vi "RX-SIM-BPCS-UDP (SubVI).vi"(8 "error in (no error)":errorcluster, 11 "UDP Network Connection in":refnum<k16>) -> (0 "error out":errorcluster, 1 "BPCS-10LI200":dbl, 2 "SIM-BPCS-RX-ARRAY":dbl[](array[numeric]), 3 "UDP Network Connection out":refnum<k16>, 5 "BPCS-10TI100":dbl)   [LabVIEW 2018]
uses:
  BPCS Global Variables.vi
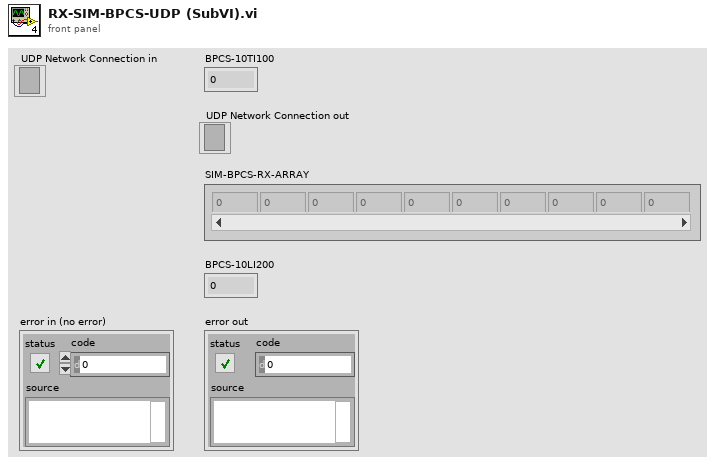
[diagram p1: front panel]
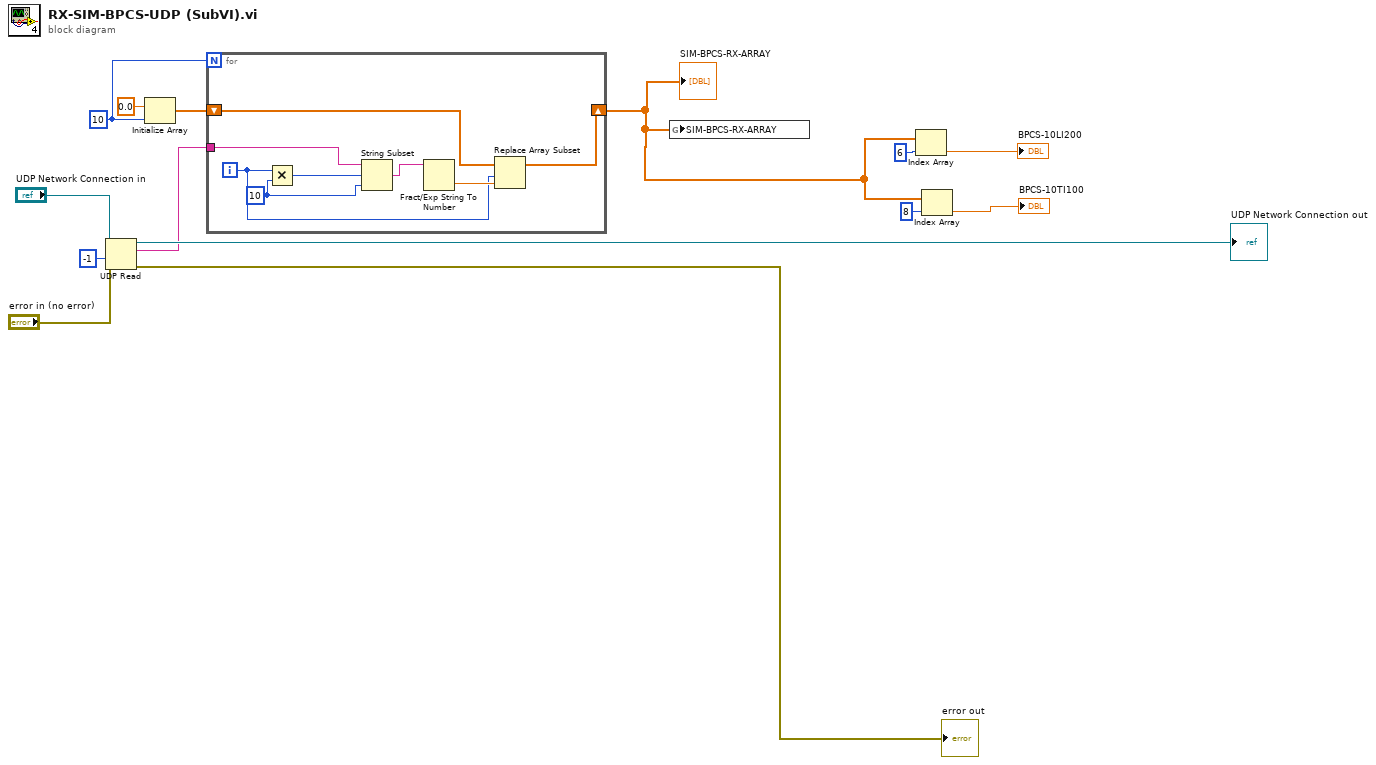
[diagram p0: block diagram]
diagram:
  w7 = 10 ("dimension size")
  n1 = UDP Read(connection ID="UDP Network Connection in", timeout ms (25000)=-1, 8:"error in (no error)") -> (data out=w3:string, error out=→"error out":errorcluster, 3:→"UDP Network Connection out":refnum<k16>)  [unwired: 3 out]
  n2 = Initialize Array(0.0 ("element"), w7) -> (w6:dbl[])
  n3 = for {
    N: w7 -> [_]
    tunnel: w3 -> [w21]
    shift-right: [w17] -> w14
    shift-left: w6 -> [w16]
    i -> [w18]
    w15 = 10 ("y")
    n4 = Multiply(x=w18, y=w15) -> (x*y=w20:i32)
    n5 = String Subset(string=w21, offset (0)=w20, length (rest)=w15) -> (substring=w22:string)
    n6 = Fract/Exp String To Number(string=w22) -> (number=w19:dbl)  [unwired: 3 in, 1 out]
    n7 = Replace Array Subset(array=w16, new element=w19, index=w18) -> (w17:dbl[])
  }
  "SIM-BPCS-RX-ARRAY" <- w14
  n8 = global write "BPCS Global Variables.vi" "SIM-BPCS-RX-ARRAY"(w14) -> ()
  n9 = Index Array(array=w14, index=6) -> (element=→"BPCS-10LI200":dbl)
  n10 = Index Array(array=w14, index=8) -> (element=→"BPCS-10TI100":dbl)
